vi "fgv_8-bit export visibility settings.vi"(8 "error in (no error)":errorcluster, 9 "Function":enum16{"Intialize", "Write", "Read", "Clear"}(ring), 10 "Include camera videos":bool, 11 "Include speed graph":bool) -> (0 "error out":errorcluster, 2 "Include camera videos":bool, 3 "Include speed graph":bool)   [LabVIEW 2017]
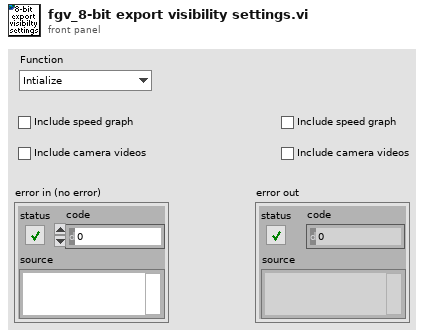
[diagram p1: front panel]
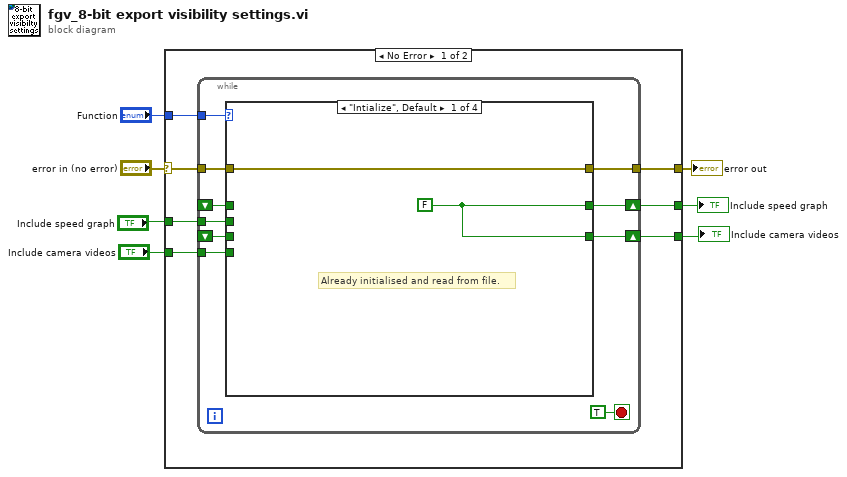
[diagram p0: block diagram]
diagram:
  n1 = case shown="No Error" "error in (no error)" {
    selector: "error in (no error)" -> [w12 w36]
    tunnel: [w13 w36] -> w6
    tunnel: "Function" -> [w14 _]
    tunnel: "Include speed graph" -> [w11 w35]
    tunnel: [w10 w35] -> w2
    tunnel: "Include camera videos" -> [w8 w34]
    tunnel: [w9 w34] -> w1
    frame No Error {
      n2 = while {
        tunnel: w14 -> [w23]
        tunnel: [w21] -> w13
        tunnel: w12 -> [w22]
        tunnel: w11 -> [w20]
        shift-right: [w19] -> w10
        shift-left: _ -> [w18]
        tunnel: w8 -> [w15]
        shift-right: [w16] -> w9
        shift-left: _ -> [w17]
        stop <- TRUE stop-if-true
        n3 = case shown="\"Intialize\", Default" w23 {
          tunnel: [w26 w29 w32 w33] -> w21
          tunnel: w22 -> [w26 w29 w32 w33]
          tunnel: w20 -> [_ w28 _ _]
          tunnel: [w25 w28 w31 _] -> w19
          tunnel: w18 -> [_ _ w31 _]
          tunnel: w15 -> [_ w27 _ _]
          tunnel: [w25 w27 w30 _] -> w16
          tunnel: w17 -> [_ _ w30 _]
          frame "Intialize", Default {
            w25 = FALSE ("Include speed graph")
            # "Already initialised and read from file."
          }
          frame "Write" {
          }
          frame "Read" {
          }
          frame "Clear" {
          }
        }
      }
    }
    frame Error {
    }
  }
  "error out" <- w6
  "Include speed graph" <- w2
  "Include camera videos" <- w1
